vi "Preset STEP HOLD time query.vi"(8 "error in (no error)":errorcluster, 11 "VISA resource in":refnum<visa-resource-name>) -> (0 "error out":errorcluster, 2 "Time":string, 3 "VISA resource out":refnum<visa-resource-name>)   [LabVIEW 2025, in "Chroma 19572.lvlib"]
doc: "This VI writes to the instrument the STEP HOLD time."
uses:
  <instrlib>/Chroma 19572/Chroma 19572.lvlib
panel:
  # "[sec]"
  # "PreSet STEP HOLD time query"
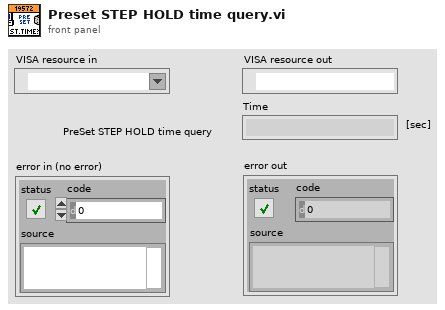
[diagram p1: front panel]
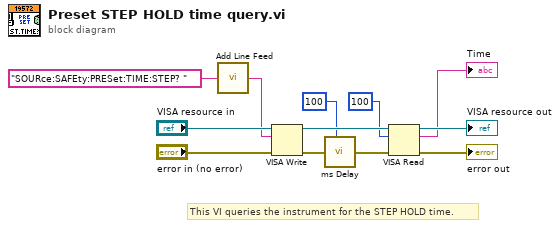
[diagram p0: block diagram]
diagram:
  # "This VI queries the instrument for the STEP HOLD time."
  n1 = call <instrlib>:"Add Line Feed.vi"("Command string"="SOURce:SAFEty:PRESet:TIME:STEP? ") -> ("Concatenated string"=w9:string)  [unwired: 4 in]
  n2 = VISA Write(VISA resource name="VISA resource in", write buffer=w9, error in (no error)="error in (no error)") -> (VISA resource name out=w12:refnum<visa-resource-name>, error out=w5:errorcluster)  [unwired: 1 out]
  n3 = call <instrlib>:"ms Delay.vi"("miliseconds to wait"=u32 100, "error in (no error)"=w5) -> ("error out"=w8:errorcluster)  [unwired: 6 in, 1 out]
  n4 = VISA Read(VISA resource name=w12, byte count=u32 100, error in (no error)=w8) -> (VISA resource name out=→"VISA resource out":refnum<visa-resource-name>, read buffer=→"Time":string, error out=→"error out":errorcluster)  [unwired: 1 out]
